vi "Set_WebService_Data.vi"(8 "error in (no error)":errorcluster, 10 "data":T1, 11 "Class in":refnum<class "AB_WebService.lvclass">) -> (0 "error out":errorcluster, 3 "Class out":refnum<class "AB_WebService.lvclass">)   [LabVIEW 2020, in "AB_WebService.lvclass"]
uses:
  <vilib>/AppBuilder/AB_Classes/WebService/AB_WebService.lvclass
  <vilib>/AppBuilder/AB_Classes/WebService/AB_WebService.ctl
  <vilib>/AppBuilder/AB_Classes/WebService/AB_WebService.lvclass/AB_WebService.ctl
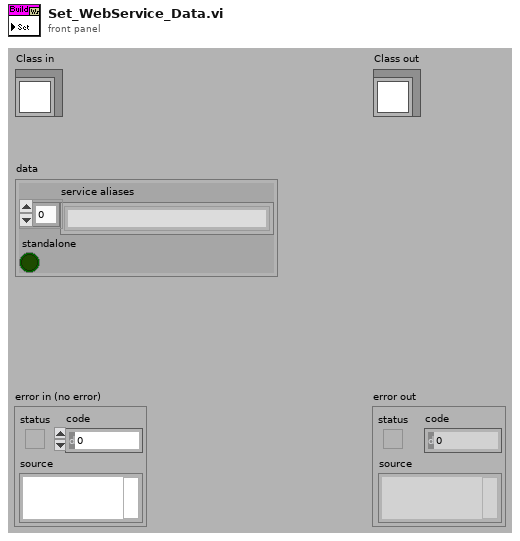
[diagram p1: front panel]
types:
  T1 = typedef "AB_WebService.ctl" = cluster{"service aliases":string[], "standalone":bool}
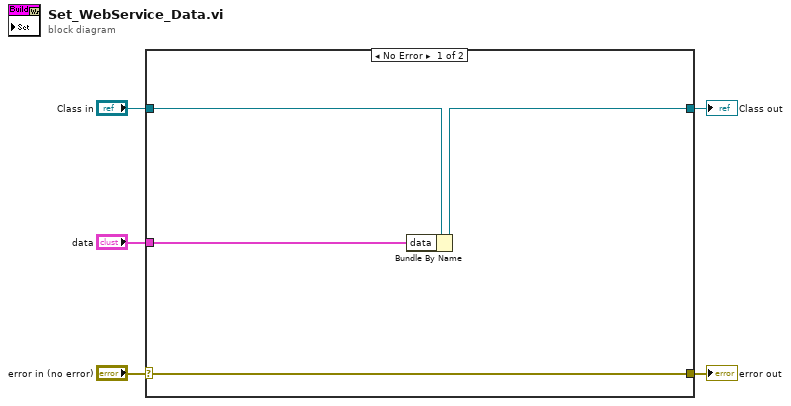
[diagram p0: block diagram]
diagram:
  n1 = case "Case" shown="No Error" "error in (no error)" {
    selector: "error in (no error)" -> [w9 w11]
    tunnel: [w9 w11] -> w4
    tunnel: [w6 w10] -> w2
    tunnel: "Class in" -> [w8 w10]
    tunnel: "data" -> [w7 _]
    frame No Error {
      n2 = Bundle By Name(cluster=w8, "data"=w7) -> (w6:refnum<class "AB_WebService.lvclass">)
    }
    frame Error {
    }
  }
  "error out" <- w4
  "Class out" <- w2
